vi "helper-do-active-verif.vi"(8 "name":string, 9 "Value":u8, 10 "State":bool, 11 "ADDR":T1 format="%04d") -> (2 "digitalPort":cluster{"State":bool, "ADDR":T1, "Timeout":u8} {"ADDR" format="%04d"}, 3 "T button?":bool)   [LabVIEW 2024]
uses:
  controls/type.address.ctl
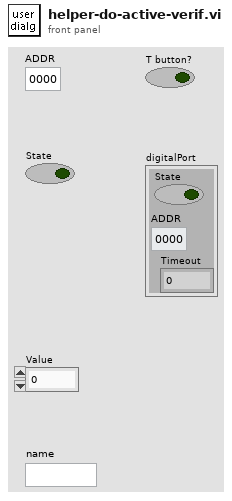
[diagram p1: front panel]
types:
  T1 = typedef "type.address.ctl" = u16
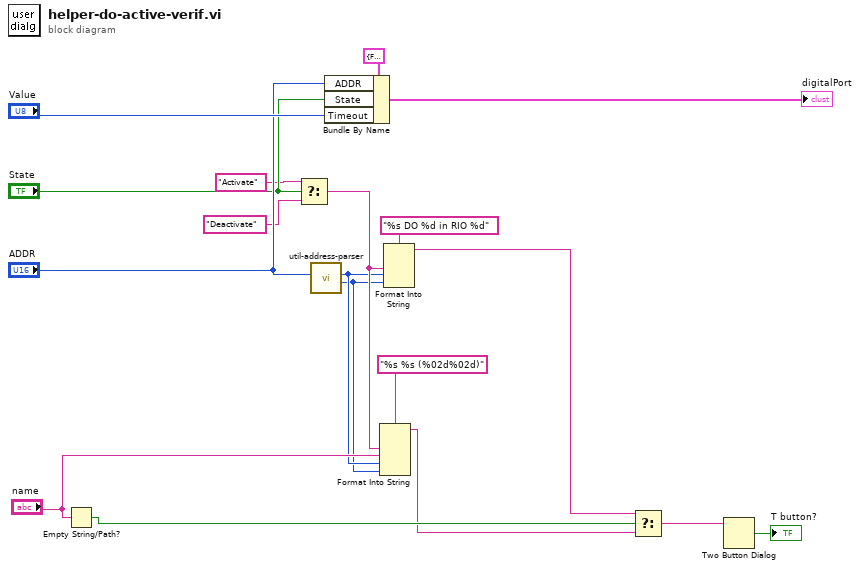
[diagram p0: block diagram]
diagram:
  n1 = Empty String/Path?(string/path="name") -> (empty?=w9:bool)
  n2 = Select(t="Activate", s="State", f="Deactivate") -> (s? t:f=w5:string)
  n3 = call "util-address-parser.vi"("ADDR 2"="ADDR") -> ("Channel"=w2:u8, "Address"=w3:u8)  [unwired: 9 in]
  n4 = Bundle By Name(cluster=cluster{"State":bool, "ADDR":T1, "Timeout":u8} {"State"=FALSE, "ADDR"=8, "Timeout"=8} ("digitalPort"), "ADDR"="ADDR", "State"="State", "Timeout"="Value") -> (→"digitalPort":cluster{"State":bool, "ADDR":T1, "Timeout":u8})
  n5 = Format Into String(format string="%s %s (%02d%02d)" ("message"), w5, "name", w3, w2) -> (resulting string=w1:string)  [unwired: 2 in, 1 out]
  n6 = Format Into String(format string="%s DO %d in RIO %d" ("message"), w5, w3, w2) -> (resulting string=w8:string)  [unwired: 2 in, 1 out]
  n7 = Select(t=w8, s=w9, f=w1) -> (s? t:f=w7:string)
  n8 = Two Button Dialog(message=w7) -> (T button?=→"T button?":bool)  [unwired: 2 in]
